vi "fill.vi"(11 "color (black)":u32) -> (3 "new picture":picture)   [LabVIEW 2023]
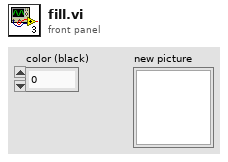
[diagram p1: front panel]
types:
  T1 = cluster{"left":i16, "top":i16, "right":i16, "bottom":i16}
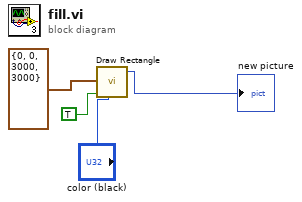
[diagram p0: block diagram]
diagram:
  n1 = call <vilib>:"Draw Rectangle.vi"("rect"=T1 {"left"=0, "top"=0, "right"=3000, "bottom"=3000}, "fill?(F)"=TRUE, "color(black)"="color (black)") -> ("new picture"=→"new picture":picture)  [unwired: 6 in]
